vi "Get pressure auto-adjust.vi"(8 "error in (no error)":errorcluster, 11 "Pressure Control in":refnum<class "Pressure Control.lvclass">) -> (0 "error out":errorcluster, 1 "Target pressure range":T1, 2 "Enabled?":bool, 3 "Pressure Control out":refnum<class "Pressure Control.lvclass">)   [LabVIEW 2011, in "Pressure Control.lvclass"]
uses:
  Pressure Control.lvclass
  Auto-adjust Pressure Range.ctl
  Pressure auto-adjust background loop.vi
  COSYLib/COSYLib.lvlib
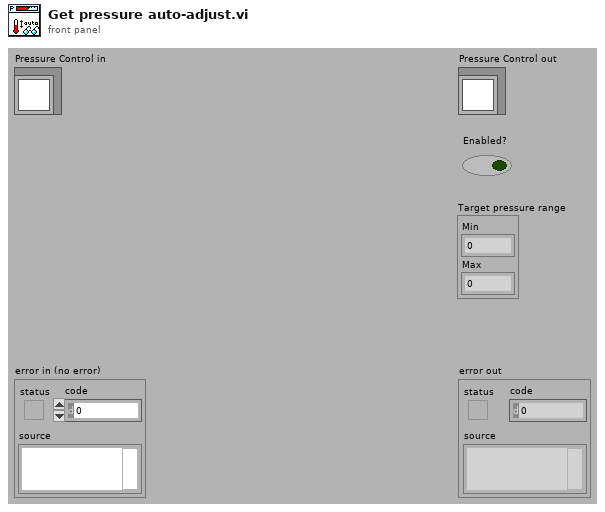
[diagram p1: front panel]
types:
  T1 = typedef "Pressure Control.lvclass/Auto-adjust Pressure Range.ctl" = cluster{"Min":dbl, "Max":dbl}
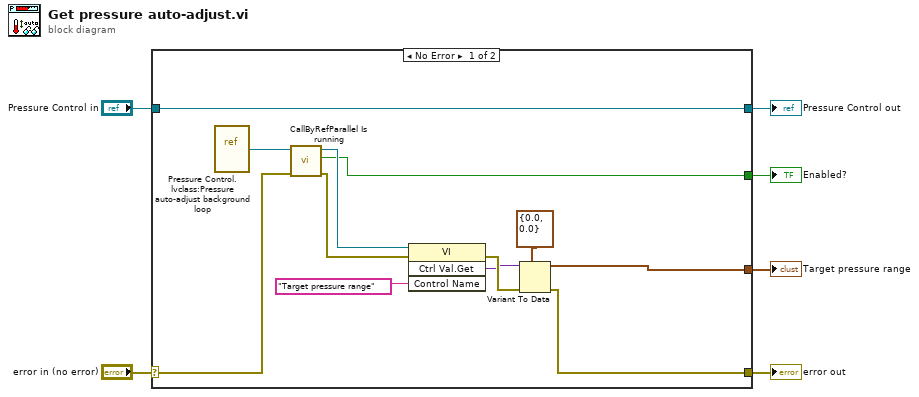
[diagram p0: block diagram]
diagram:
  n1 = case shown="No Error" "error in (no error)" {
    selector: "error in (no error)" -> [w8 w20]
    tunnel: [w11 w20] -> w5
    tunnel: [w16 w19] -> w3
    tunnel: "Pressure Control in" -> [w16 w19]
    tunnel: [w9 _] -> w2
    tunnel: [w12 _] -> w1
    frame No Error {
      n2 = vi-ref "Pressure Control.lvclass:Pressure auto-adjust background loop.vi"() -> (w10:refnum<vi>)
      n3 = call "CallByRefParallel Is running.vi"("error in (no error)"=w8, "VI Refnum"=w10) -> ("error out"=w7:errorcluster, "Is running?"=w9:bool, "VI Refnum dup"=w18:refnum<vi>)  [unwired: 7 in]
      n4 = invoke class="VI" method="Ctrl Val.Get"(reference=w18, error in=w7, "Control Name"="Target pressure range") -> (error out=w17:errorcluster, "Get Control Value Variant"=w14:variant)  [unwired: 1 in, 2 out]
      n5 = Variant To Data(error in=w17, type=T1 {"Min"=0.0, "Max"=0.0} ("Target pressure range"), Variant=w14) -> (data=w12:T1, error out=w11:errorcluster)
    }
    frame Error {
    }
  }
  "error out" <- w5
  "Pressure Control out" <- w3
  "Enabled?" <- w2
  "Target pressure range" <- w1
